vi "Periodic Tasks.vi"   [LabVIEW 2014]
doc: "This VI runs in parallel to other tasks. It can contain as many user-defined periodic loops as you need. These can carry out PID or other sorts of timed response."
uses:
  Robot Global Data.vi
  <vilib>/Rock Robotics/Network Tables/SD Write Number.vi
types:
  T1 = cluster{"Lift":cluster{"Top":bool, "High":bool, "Mid":bool, "Low":bool, "Bot":bool}, "Clamp":cluster{"Widest":bool, "Shortest":bool, "Tote 1":bool, "Tote 2":bool}, "Tote Detected":bool}
  T2 = cluster{"Top":bool, "High":bool, "Mid":bool, "Low":bool, "Bot":bool}
  T3 = cluster{"Widest":bool, "Shortest":bool, "Tote 1":bool, "Tote 2":bool}
  T4 = cluster{"Limit Switches":cluster{"Lift":cluster{"Top":bool, "High":bool, "Mid":bool, "Low":bool, "Bot":bool}, "Clamp":cluster{"Widest":bool, "Shortest":bool, "Tote 1":bool, "Tote 2":bool}, "Tote Detected":bool}, "Distance (in)":dbl, "Clamp Wide":bool, "Lift Distance":dbl}
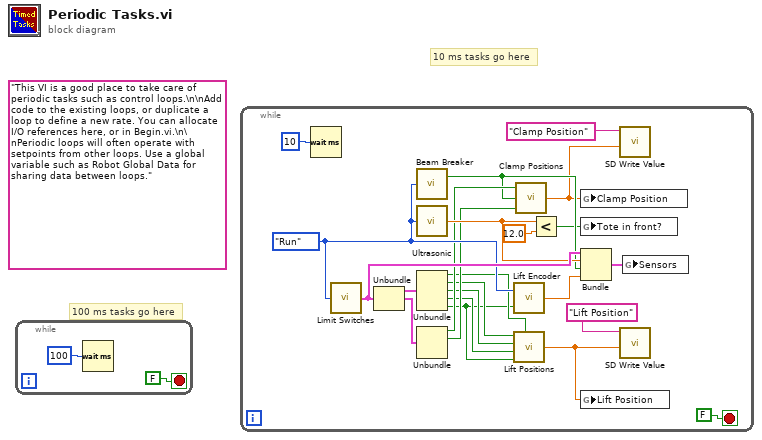
[diagram p0: block diagram]
diagram:
  (unwired) "This VI is a good place to take care of periodic tasks such as control loops.\n\nAdd code to the existing loops, or duplicate a loop to define a new rate. You can allocate I/O references here, or in Begin.vi.\n\nPeriodic loops will often operate with setpoints from other loops. Use a global variable such as Robot Global Data for sharing data between loops."
  # "100 ms tasks go here"
  # "10 ms tasks go here"
  n1 = while {
    stop <- FALSE stop-if-true
    n2 = Wait (ms)(milliseconds to wait=u32 100) -> ()  [unwired: 1 out]
  }
  n3 = while {
    stop <- FALSE stop-if-true
    w20 = enum8{"Start", "Run", "Finish"}."Run" ("Mode")
    n4 = Wait (ms)(milliseconds to wait=u32 10) -> ()  [unwired: 1 out]
    n5 = call "Limit Switches.vi"("Mode"=w20) -> ("Limit Switches"=w21:T1)
    n6 = Unbundle(w21) -> ("Lift"=w23:T2, "Clamp"=w22:T3)  [unwired: 1 out]
    n7 = call "Beam Breaker.vi"("Mode"=w20) -> ("Clamp Wide"=w14:bool)  [unwired: 1 in]
    n8 = call "Ultrasonic.vi"("Mode"=w20) -> ("Distance (in)"=w17:dbl)
    n9 = Unbundle(w23) -> ("Top"=w12:bool, "High"=w11:bool, "Mid"=w10:bool, "Low"=w9:bool, "Bot"=w6:bool)
    n10 = Unbundle(w22) -> ("Widest"=w15:bool, "Shortest"=w13:bool)  [unwired: 2 out]
    n11 = call "Lift Encoder.vi"("Reset"=w6, "Mode"=w20) -> ("Lift Distance"=w5:dbl)
    n12 = call "Lift Positions.vi"("High"=w11, "Middle"=w10, "Low"=w9, "Bottom"=w6, "Top"=w12) -> ("Clamp Position"=w7:dbl)
    n13 = call "Clamp Positions.vi"("Shortest (LS)"=w13, "Wide (BB)"=w14, "Widest (LS)"=w15) -> ("Clamp Position"=w8:dbl)
    n14 = Less?(x=w17, y=12.0) -> (x < y?=w3:bool)
    n15 = global write "Robot Global Data.vi" "Clamp Position"(w8) -> ()
    n16 = global write "Robot Global Data.vi" "Tote in front?"(w3) -> ()
    n17 = Bundle("Limit Switches"=w21, "Distance (in)"=w17, "Clamp Wide"=w14, "Lift Distance"=w5) -> (w4:T4)  [unwired: 1 in]
    n18 = global write "Robot Global Data.vi" "Lift Position"(w7) -> ()
    n19 = call-poly <vilib>:"SD Write Value.vi"("Numeric"=w8, "Name"="Clamp Position") -> ()  [unwired: 8 in, 2 out]
    n20 = call-poly <vilib>:"SD Write Value.vi"("Numeric"=w7, "Name"="Lift Position") -> ()  [unwired: 8 in, 2 out]
    n21 = global write "Robot Global Data.vi" "Sensors"(w4) -> ()
  }
